vi "Read_async_master_PN.vi"(0 "master N channels":u32, 1 "master buffer size":i32, 2 "master task in":i32, 11 "Samples Per Channel":i32=-1, 12 "Timeout":dbl=10.0) -> (4 "master task out":i32, 8 "master data":dbl[][](array[numeric]), 15 "error out":errorcluster)   [LabVIEW 2011]
uses:
  <userlib>/LV-Link3/PolySubVIs/DtOLReadMultiple2D.vi
  <userlib>/LV-Link3/PolySubVIs/DtOLStartNormal.vi
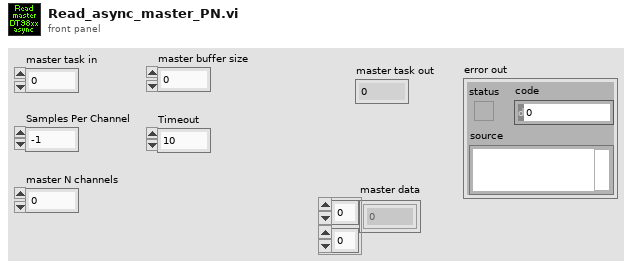
[diagram p1: front panel]
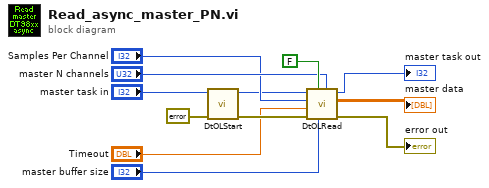
[diagram p0: block diagram]
diagram:
  n1 = call-poly <userlib>:"DtOLStart.vi"("error in (no error)"=errorcluster {"status"=FALSE, "code"=0, "source"=""}, "Task in"="master task in") -> ("error out"=w2:errorcluster, "Task out"=w4:i32)  [unwired: 8 in]
  n2 = call-poly <userlib>:"DtOLRead.vi"("Number Chan to Read"="master N channels", "Buffer size"="master buffer size", "OnlyReadAvailable"=FALSE, "error in (no error)"=w2, "Timeout"="Timeout", "Samples Per Channel"="Samples Per Channel", "Task in"=w4) -> ("error out"=→"error out":errorcluster, "2D Data out"=→"master data":dbl[][], "Task out"=→"master task out":i32)  [unwired: 2 out]
